vi "Init.vi"(8 "error in (no error)":errorcluster, 11 "Data in":refnum<class "FPGA-Bus.lvclass">) -> (0 "error out":errorcluster, 3 "Data out":refnum<class "FPGA-Bus.lvclass">)   [LabVIEW 2021, in "FPGA-Bus.lvclass"]
doc: "Abstract Data Classes 2.1.1.12\nTim Streeter - TSA\nCopyright (c) 2024, TSAOmni-Bus 2.0.1.6\nTim - TSA\nCopyright (c) 2024, TSA"
uses:
  FPGA-Bus.lvclass
  C:/Program Files (x86)/National Instruments/LabVIEW 2021/vi.lib/TSA/Omni-Bus/Omni-Bus/Bus Access/Bus_Access.lvclass
  <vilib>/TSA/Omni-Bus/Omni-Bus/Bus Access/Bus_Access.lvclass/Bus_Access.ctl
  FPGA-Bus.lvclass/FPGA-Bus.ctl
  Support/Boolean/FPGA-Bus_Boolean.lvclass
  C:/Program Files (x86)/National Instruments/LabVIEW 2021/vi.lib/TSA/Abstract Data Classes/Abs_Types/Value/Abs_Value.lvclass
  Support/Boolean/FPGA-Bus_Boolean.lvclass/FPGA-Bus_Boolean.ctl
  Support/SGL/FPGA-Bus_SGL.lvclass
  Support/SGL/Support/FPGA Type.ctl
  Support/SGL/FPGA-Bus_SGL.lvclass/FPGA-Bus_SGL.ctl
  Support/I8/Support/FPGA Type.ctl
  Support/I8/FPGA-Bus_I8.lvclass
  Support/I8/FPGA-Bus_I8.lvclass/FPGA-Bus_I8.ctl
  Support/I16/Support/FPGA Type.ctl
  Support/I16/FPGA-Bus_I16.lvclass
  Support/I16/FPGA-Bus_I16.lvclass/FPGA-Bus_I16.ctl
  Support/I32/Support/FPGA Type.ctl
  Support/I32/FPGA-Bus_I32.lvclass
  Support/I32/FPGA-Bus_I32.lvclass/FPGA-Bus_I32.ctl
  Support/I64/Support/FPGA Type.ctl
  Support/I64/FPGA-Bus_I64.lvclass
  Support/I64/FPGA-Bus_I64.lvclass/FPGA-Bus_I64.ctl
  Support/U8/Support/FPGA Type.ctl
  Support/U8/FPGA-Bus_U8.lvclass
  Support/U8/FPGA-Bus_U8.lvclass/FPGA-Bus_U8.ctl
  Support/U16/Support/FPGA Type.ctl
  Support/U16/FPGA-Bus_U16.lvclass
  Support/U16/FPGA-Bus_U16.lvclass/FPGA-Bus_U16.ctl
  Support/U32/Support/FPGA Type.ctl
  Support/U32/FPGA-Bus_U32.lvclass
  Support/U32/FPGA-Bus_U32.lvclass/FPGA-Bus_U32.ctl
  Support/U64/Support/FPGA Type.ctl
  Support/U64/FPGA-Bus_U64.lvclass
  Support/U64/FPGA-Bus_U64.lvclass/FPGA-Bus_U64.ctl
  Support/FXP20_5/Support/FPGA Type.ctl
  Support/FXP20_5/FPGA-Bus_FXP20_5.lvclass
  C:/Program Files (x86)/National Instruments/LabVIEW 2021/vi.lib/TSA/Abstract Data Classes/Abs_Types/Double Float/Abs_Double Float.lvclass
  Support/FXP20_5/FPGA-Bus_FXP20_5.lvclass/FPGA-Bus_FXP20_5.ctl
  Support/FXP24_-2/Support/FPGA Type.ctl
  Support/FXP24_-2/FPGA-Bus_FXP24_-2.lvclass
  Support/FXP24_-2/FPGA-Bus_FXP24_-2.lvclass/FPGA-Bus_FXP24_-2.ctl
  Support/FXP24_5/Support/FPGA Type.ctl
  Support/FXP24_5/FPGA-Bus_FXP24_5.lvclass
  Support/FXP24_5/FPGA-Bus_FXP24_5.lvclass/FPGA-Bus_FXP24_5.ctl
  Support/FXP24_10/Support/FPGA Type.ctl
  Support/FXP24_10/FPGA-Bus_FXP24_10.lvclass
  Support/FXP24_10/FPGA-Bus_FXP24_10.lvclass/FPGA-Bus_FXP24_10.ctl
  Support/FXP16_3/Support/FPGA Type.ctl
  Support/FXP16_3/FPGA-Bus_FXP16_3.lvclass
  Support/FXP16_3/FPGA-Bus_FXP16_3.lvclass/FPGA-Bus_FXP16_3.ctl
  Support/FXP18_3/Support/FPGA Type.ctl
  Support/FXP18_3/FPGA-Bus_FXP18_3.lvclass
  Support/FXP18_3/FPGA-Bus_FXP18_3.lvclass/FPGA-Bus_FXP18_3.ctl
  <vilib>/NI/LVFPGA Adv Session Resources/OpenByNameSubVI.vi
  Support/Boolean/Properties/Write FPGA Interface.vi
  Support/SGL/Properties/Write FPGA Interface.vi
  Support/I8/Properties/Write FPGA Interface.vi
  Support/I16/Properties/Write FPGA Interface.vi
  Support/I32/Properties/Write FPGA Interface.vi
  Support/I64/Properties/Write FPGA Interface.vi
  Support/U8/Properties/Write FPGA Interface.vi
  Support/U16/Properties/Write FPGA Interface.vi
  Support/U32/Properties/Write FPGA Interface.vi
  Support/U64/Properties/Write FPGA Interface.vi
  Support/FXP20_5/Properties/Write FPGA Interface.vi
  Support/FXP24_-2/Properties/Write FPGA Interface.vi
  Support/FXP24_5/Properties/Write FPGA Interface.vi
  Support/FXP24_10/Properties/Write FPGA Interface.vi
  Support/FXP16_3/Properties/Write FPGA Interface.vi
  Support/FXP18_3/Properties/Write FPGA Interface.vi
  <vilib>/TSA/Omni-Bus/Omni-Bus/Bus Access/Properties/Read Tag Root.vi
  <vilib>/TSA/Omni-Bus/Omni-Bus/Bus Access/Properties/Write Values.vi
  <vilib>/TSA/Omni-Bus/Omni-Bus/Bus Access/Properties/Write Tags.vi
  <vilib>/TSA/Abstract Data Classes/Abs_Types/Double Float/Abs_Double Float.lvclass
  <vilib>/TSA/Abstract Data Classes/Abs_Types/Value/Abs_Value.lvclass
  C:/Program Files (x86)/National Instruments/LabVIEW 2021/vi.lib/TSA/Abstract Data Classes/Abs_Types/Type/Abs_Type.lvclass
  <vilib>/rvi/interface/common/dynamic/niFpgaEscapeDelimiterAndNull.vi
  <vilib>/Utility/error.llb/Error Cluster From Error Code.vi
  <vilib>/NI/LVFPGA Adv Session Resources/OpenByName.xnode
  <vilib>/NI/LVFPGA Adv Session Resources/LVFPGAAdvSessionResources.lvlib
  <vilib>/Utility/Data Type/NI_Data Type.lvlib
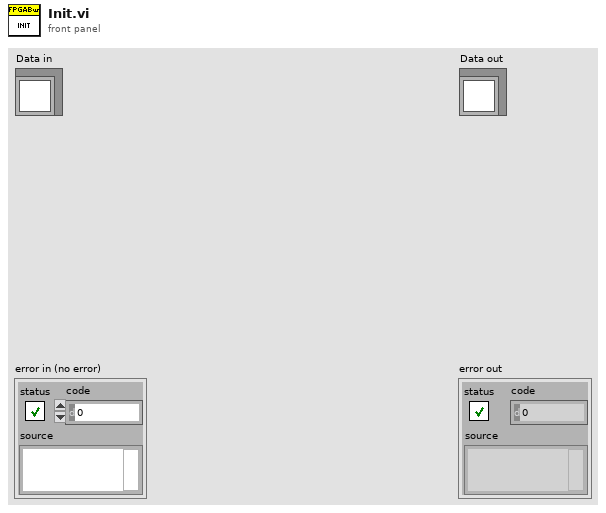
[diagram p1: front panel]
types:
  T1 = typedef "LVFPGAAdvSessionResources.lvlib/ResourceInfo.ctl" = cluster{"Resource name":string, "Data type":variant, "Resource type":enum16{"Register", "Host To Target FIFO", "Target To Host FIFO"}}
  T2 = cluster{"Name":string, "Depth":u32, "Write? (Deprecated:Use Implementation)":bool, "Physical Channel":u32, "Base Address":u32, "Data Width":u32, "Data Type":enum32{"Boolean", "I8", "I16", "I32", "I64", "U8", "U16", "U32", "U64", "FXP", "CustomControl", "SGL"}, "FXP Properties":variant, "Write Window Address":u32, "Implementation":enum16{"niFpgaTargetToHost", "niFpgaHostToTarget", "niFpgaPeerToPeerWriter", "niFpgaPeerToPeerReader", "niCoreTargetToHost", "niCoreHostToTarget"}, "Control Set":u32}[]
  T3 = cluster{"Name":string, "type":variant, "indicator?":bool}[]
  T4 = typedef "FPGA-Bus_SGL.lvclass/FPGA Type.ctl" = refnum<k20>
  T5 = typedef "FPGA-Bus_I8.lvclass/FPGA Type.ctl" = refnum<k20>
  T6 = typedef "FPGA-Bus_I16.lvclass/FPGA Type.ctl" = refnum<k20>
  T7 = typedef "FPGA-Bus_I32.lvclass/FPGA Type.ctl" = refnum<k20>
  T8 = typedef "FPGA-Bus_I64.lvclass/FPGA Type.ctl" = refnum<k20>
  T9 = typedef "FPGA-Bus_U8.lvclass/FPGA Type.ctl" = refnum<k20>
  T10 = typedef "FPGA-Bus_U16.lvclass/FPGA Type.ctl" = refnum<k20>
  T11 = typedef "FPGA-Bus_U32.lvclass/FPGA Type.ctl" = refnum<k20>
  T12 = typedef "FPGA-Bus_U64.lvclass/FPGA Type.ctl" = refnum<k20>
  T13 = typedef "FPGA-Bus_FXP20_5.lvclass/FPGA Type.ctl" = refnum<k20>
  T14 = typedef "FPGA-Bus_FXP24_-2.lvclass/FPGA Type.ctl" = refnum<k20>
  T15 = typedef "FPGA-Bus_FXP24_5.lvclass/FPGA Type.ctl" = refnum<k20>
  T16 = typedef "FPGA-Bus_FXP24_10.lvclass/FPGA Type.ctl" = refnum<k20>
  T17 = typedef "FPGA-Bus_FXP16_3.lvclass/FPGA Type.ctl" = refnum<k20>
  T18 = typedef "FPGA-Bus_FXP18_3.lvclass/FPGA Type.ctl" = refnum<k20>
  T19 = typedef "NI_Data Type.lvlib/Data Type.ctl" = enum8{"Invalid Type", "Void", "I8", "I16", "I32", "I64", "U8", "U16", "U32", "U64", "Single Float", "Double Float", "Extended Float", "Single Complex", "Double Complex", "Extended Complex", "Enum U8", "Enum U16", "Enum U32", "Enum U64", "Single Float With Unit", "Double Float With Unit", "Extended Float With Unit", "Single Complex with Unit", "Double Complex with Unit", "Extended Complex with Unit", "Boolean", "String", "Path", "Picture", "Tag", "Array", "Cluster", "Variant", "LV Variant", "Waveform", "Timestamp", "Digital Waveform", "Digital Data", "ExpressData", "Refnum", "External Data", "VI", "Poly VI", "LabVIEW Class Instance", "Fixed Point", "Set Collection", "Map Collection"}
  T20 = typedef "LVFixedPointRepBitsTypeDef.ctl" = cluster{"Signed":bool, "Word Length":u32, "Integer Word Length":i32}
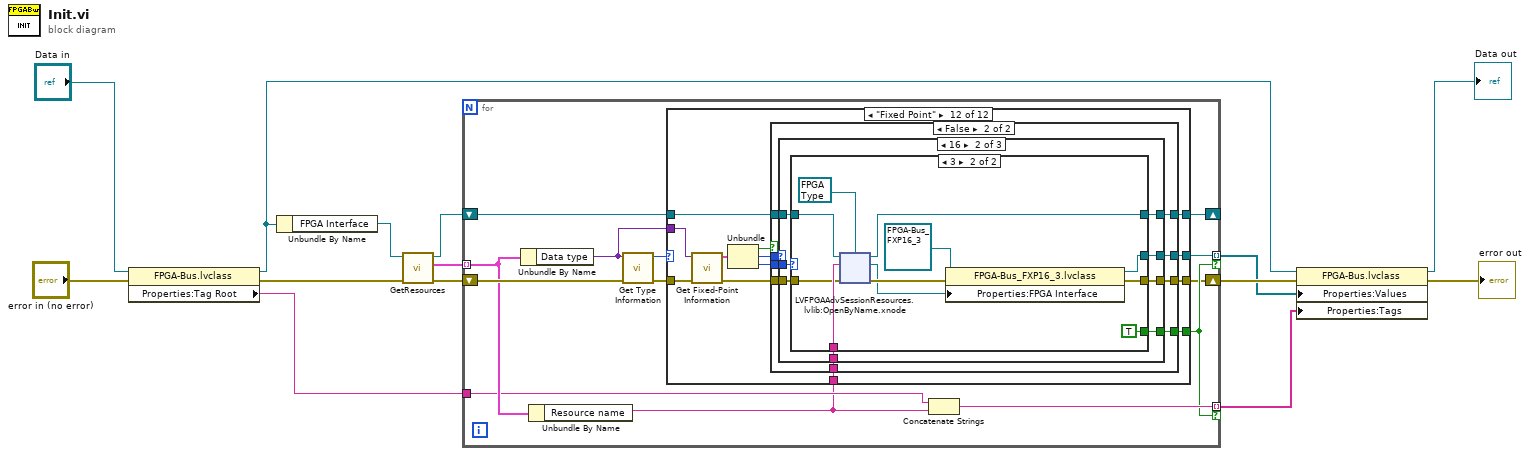
[diagram p0: block diagram]
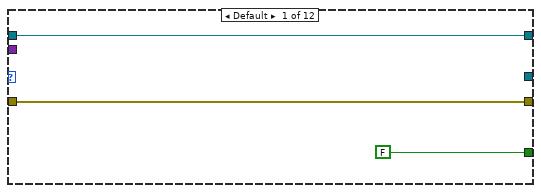
[diagram p2: hidden frame]
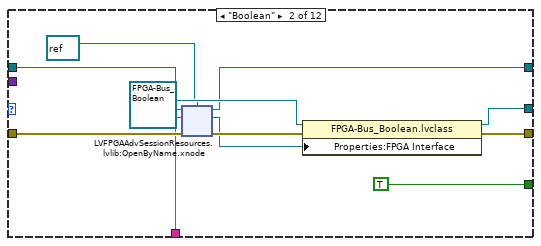
[diagram p3: hidden frame]
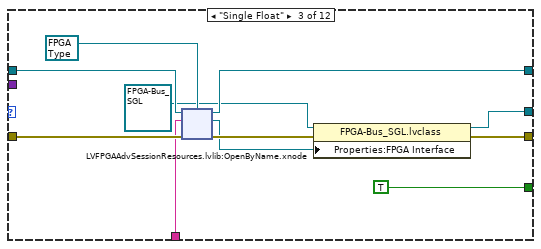
[diagram p4: hidden frame]
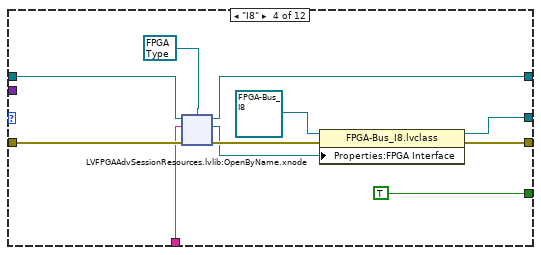
[diagram p5: hidden frame]
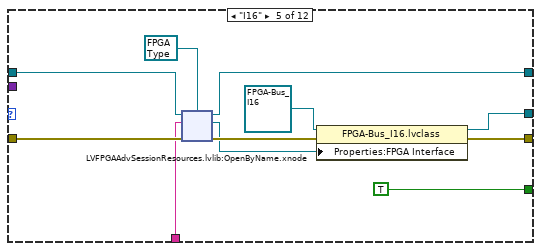
[diagram p6: hidden frame]
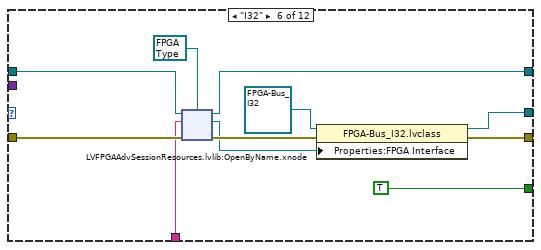
[diagram p7: hidden frame]
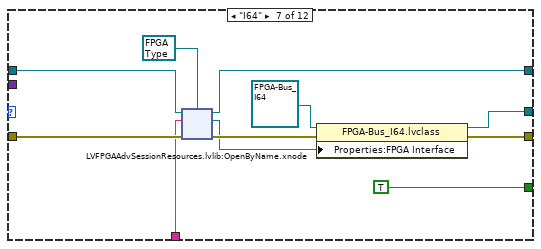
[diagram p8: hidden frame]
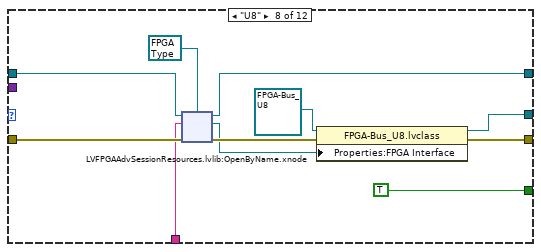
[diagram p9: hidden frame]
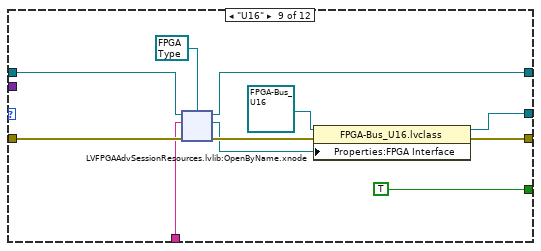
[diagram p10: hidden frame]
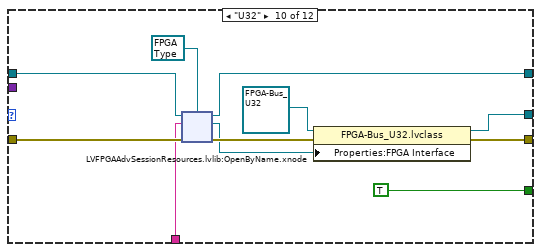
[diagram p11: hidden frame]
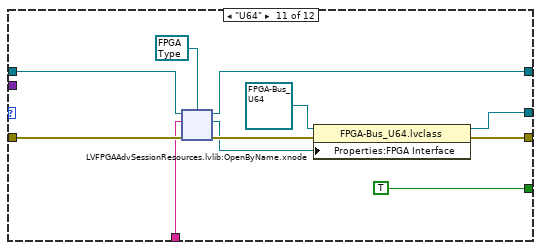
[diagram p12: hidden frame]
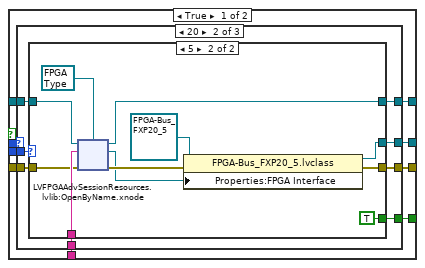
[diagram p13: hidden frame]
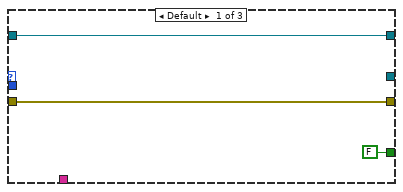
[diagram p14: hidden frame]
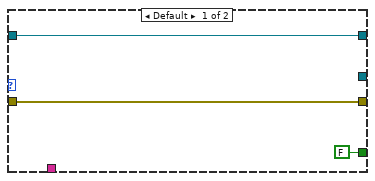
[diagram p15: hidden frame]
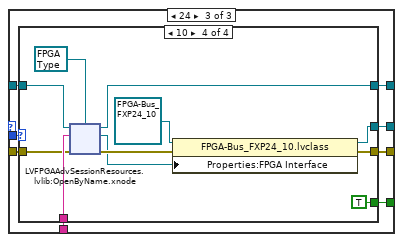
[diagram p16: hidden frame]
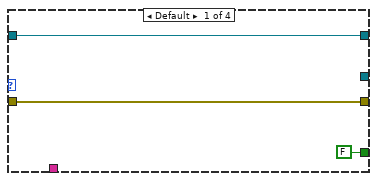
[diagram p17: hidden frame]
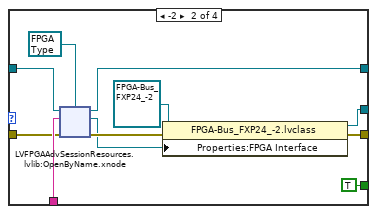
[diagram p18: hidden frame]
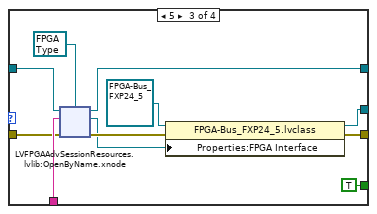
[diagram p19: hidden frame]
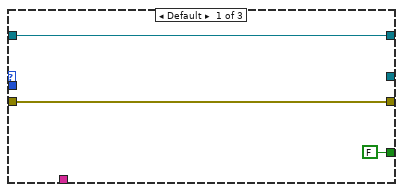
[diagram p20: hidden frame]
diagram:
  n1 = property class="FPGA-Bus.lvclass"(reference="Data in", error in="error in (no error)") -> (reference out=w5:refnum<class "FPGA-Bus.lvclass">, error out=w7:errorcluster, "Properties:Tag Root"=w8:string)
  n2 = Unbundle By Name(w5) -> ("FPGA Interface"=w14:refnum<k20>)
  n3 = call <vilib>:"GetResources.vi"("error in (no error)"=w7, "FPGA VI Reference in"=w14) -> ("error out"=w13:errorcluster, "Resource info out"=w12:T1[], "FPGA VI Reference out"=w11:refnum<k20>)  [unwired: 7 in]
  n4 = for {
    shift-right: [w19] -> w6
    shift-left: w13 -> [w27]
    tunnel: w12 -> [w25] mode=indexing
    tunnel: [w23] -> w4 mode=indexing if=w21
    shift-right: [w16] -> _
    shift-left: w11 -> [w17]
    tunnel: w8 -> [w24]
    tunnel: [w22] -> w1 mode=indexing if=w21
    n5 = Unbundle By Name(w25) -> ("Data type"=w15:variant)
    n6 = Unbundle By Name(w25) -> ("Resource name"=w18:string)
    n7 = call <vilib>:"Get Type Information.vi"("error in (no error)"=w27, "variant"=w15) -> ("error out"=w20:errorcluster, "type"=w26:T19)  [unwired: 5 in, 3 out]
    n8 = case shown="\"Fixed Point\"" w26 {
      tunnel: [FALSE TRUE TRUE TRUE TRUE TRUE TRUE TRUE TRUE TRUE TRUE w283] -> w21
      tunnel: [_ w39 w64 w88 w112 w136 w160 w184 w208 w232 w256 w282] -> w22
      tunnel: w20 -> [w29 w37 w62 w86 w110 w134 w158 w182 w206 w230 w254 w277]
      tunnel: [w29 w38 w63 w87 w111 w135 w159 w183 w207 w231 w255 w281] -> w19
      tunnel: w18 -> [_ w36 w61 w85 w109 w133 w157 w181 w205 w229 w253 w280]
      tunnel: w17 -> [w30 w35 w60 w84 w108 w132 w156 w180 w204 w228 w252 w279]
      tunnel: [w30 w34 w59 w83 w107 w131 w155 w179 w203 w227 w251 w278] -> w16
      tunnel: w15 -> [_ _ _ _ _ _ _ _ _ _ _ w276]
      frame Default {
      }
      frame "Boolean" {
        n9 = xnode "LVFPGAAdvSessionResources.lvlib:OpenByName.xnode"("FPGA VI Reference in"=w35, "Resource name in"=w36, "Single resource reference type in"=refnum<k20> refnum ("FPGA Interface"), "Error in"=w37) -> ("Single resource reference out"=w31:refnum<k20>, "Error out"=w33:errorcluster, "FPGA VI Reference out"=w34:refnum<k20>)
        n10 = property class="FPGA-Bus_Boolean.lvclass"(reference=refnum<class "FPGA-Bus_Boolean.lvclass"> refnum ("FPGA-Bus_Boolean.lvclass"), error in=w33, "Properties:FPGA Interface"=w31) -> (reference out=w39:refnum<class "FPGA-Bus_Boolean.lvclass">, error out=w38:errorcluster)
      }
      frame "Single Float" {
        n11 = xnode "LVFPGAAdvSessionResources.lvlib:OpenByName.xnode"("FPGA VI Reference in"=w60, "Resource name in"=w61, "Single resource reference type in"=T4 refnum ("FPGA Interface"), "Error in"=w62) -> ("Single resource reference out"=w55:T4, "Error out"=w58:errorcluster, "FPGA VI Reference out"=w59:refnum<k20>)
        n12 = property class="FPGA-Bus_SGL.lvclass"(reference=refnum<class "FPGA-Bus_SGL.lvclass"> refnum ("FPGA-Bus_SGL.lvclass"), error in=w58, "Properties:FPGA Interface"=w55) -> (reference out=w64:refnum<class "FPGA-Bus_SGL.lvclass">, error out=w63:errorcluster)
      }
      frame "I8" {
        n13 = xnode "LVFPGAAdvSessionResources.lvlib:OpenByName.xnode"("FPGA VI Reference in"=w84, "Resource name in"=w85, "Single resource reference type in"=T5 refnum ("FPGA Interface"), "Error in"=w86) -> ("Single resource reference out"=w81:T5, "Error out"=w82:errorcluster, "FPGA VI Reference out"=w83:refnum<k20>)
        n14 = property class="FPGA-Bus_I8.lvclass"(reference=refnum<class "FPGA-Bus_I8.lvclass"> refnum ("FPGA-Bus_I8.lvclass"), error in=w82, "Properties:FPGA Interface"=w81) -> (reference out=w88:refnum<class "FPGA-Bus_I8.lvclass">, error out=w87:errorcluster)
      }
      frame "I16" {
        n15 = xnode "LVFPGAAdvSessionResources.lvlib:OpenByName.xnode"("FPGA VI Reference in"=w108, "Resource name in"=w109, "Single resource reference type in"=T6 refnum ("FPGA Interface"), "Error in"=w110) -> ("Single resource reference out"=w105:T6, "Error out"=w106:errorcluster, "FPGA VI Reference out"=w107:refnum<k20>)
        n16 = property class="FPGA-Bus_I16.lvclass"(reference=refnum<class "FPGA-Bus_I16.lvclass"> refnum ("FPGA-Bus_I16.lvclass"), error in=w106, "Properties:FPGA Interface"=w105) -> (reference out=w112:refnum<class "FPGA-Bus_I16.lvclass">, error out=w111:errorcluster)
      }
      frame "I32" {
        n17 = xnode "LVFPGAAdvSessionResources.lvlib:OpenByName.xnode"("FPGA VI Reference in"=w132, "Resource name in"=w133, "Single resource reference type in"=T7 refnum ("FPGA Interface"), "Error in"=w134) -> ("Single resource reference out"=w129:T7, "Error out"=w130:errorcluster, "FPGA VI Reference out"=w131:refnum<k20>)
        n18 = property class="FPGA-Bus_I32.lvclass"(reference=refnum<class "FPGA-Bus_I32.lvclass"> refnum ("FPGA-Bus_I32.lvclass"), error in=w130, "Properties:FPGA Interface"=w129) -> (reference out=w136:refnum<class "FPGA-Bus_I32.lvclass">, error out=w135:errorcluster)
      }
      frame "I64" {
        n19 = xnode "LVFPGAAdvSessionResources.lvlib:OpenByName.xnode"("FPGA VI Reference in"=w156, "Resource name in"=w157, "Single resource reference type in"=T8 refnum ("FPGA Interface"), "Error in"=w158) -> ("Single resource reference out"=w153:T8, "Error out"=w154:errorcluster, "FPGA VI Reference out"=w155:refnum<k20>)
        n20 = property class="FPGA-Bus_I64.lvclass"(reference=refnum<class "FPGA-Bus_I64.lvclass"> refnum ("FPGA-Bus_I64.lvclass"), error in=w154, "Properties:FPGA Interface"=w153) -> (reference out=w160:refnum<class "FPGA-Bus_I64.lvclass">, error out=w159:errorcluster)
      }
      frame "U8" {
        n21 = xnode "LVFPGAAdvSessionResources.lvlib:OpenByName.xnode"("FPGA VI Reference in"=w180, "Resource name in"=w181, "Single resource reference type in"=T9 refnum ("FPGA Interface"), "Error in"=w182) -> ("Single resource reference out"=w177:T9, "Error out"=w178:errorcluster, "FPGA VI Reference out"=w179:refnum<k20>)
        n22 = property class="FPGA-Bus_U8.lvclass"(reference=refnum<class "FPGA-Bus_U8.lvclass"> refnum ("FPGA-Bus_U8.lvclass"), error in=w178, "Properties:FPGA Interface"=w177) -> (reference out=w184:refnum<class "FPGA-Bus_U8.lvclass">, error out=w183:errorcluster)
      }
      frame "U16" {
        n23 = xnode "LVFPGAAdvSessionResources.lvlib:OpenByName.xnode"("FPGA VI Reference in"=w204, "Resource name in"=w205, "Single resource reference type in"=T10 refnum ("FPGA Interface"), "Error in"=w206) -> ("Single resource reference out"=w201:T10, "Error out"=w202:errorcluster, "FPGA VI Reference out"=w203:refnum<k20>)
        n24 = property class="FPGA-Bus_U16.lvclass"(reference=refnum<class "FPGA-Bus_U16.lvclass"> refnum ("FPGA-Bus_U16.lvclass"), error in=w202, "Properties:FPGA Interface"=w201) -> (reference out=w208:refnum<class "FPGA-Bus_U16.lvclass">, error out=w207:errorcluster)
      }
      frame "U32" {
        n25 = xnode "LVFPGAAdvSessionResources.lvlib:OpenByName.xnode"("FPGA VI Reference in"=w228, "Resource name in"=w229, "Single resource reference type in"=T11 refnum ("FPGA Interface"), "Error in"=w230) -> ("Single resource reference out"=w225:T11, "Error out"=w226:errorcluster, "FPGA VI Reference out"=w227:refnum<k20>)
        n26 = property class="FPGA-Bus_U32.lvclass"(reference=refnum<class "FPGA-Bus_U32.lvclass"> refnum ("FPGA-Bus_U32.lvclass"), error in=w226, "Properties:FPGA Interface"=w225) -> (reference out=w232:refnum<class "FPGA-Bus_U32.lvclass">, error out=w231:errorcluster)
      }
      frame "U64" {
        n27 = xnode "LVFPGAAdvSessionResources.lvlib:OpenByName.xnode"("FPGA VI Reference in"=w252, "Resource name in"=w253, "Single resource reference type in"=T12 refnum ("FPGA Interface"), "Error in"=w254) -> ("Single resource reference out"=w249:T12, "Error out"=w250:errorcluster, "FPGA VI Reference out"=w251:refnum<k20>)
        n28 = property class="FPGA-Bus_U64.lvclass"(reference=refnum<class "FPGA-Bus_U64.lvclass"> refnum ("FPGA-Bus_U64.lvclass"), error in=w250, "Properties:FPGA Interface"=w249) -> (reference out=w256:refnum<class "FPGA-Bus_U64.lvclass">, error out=w255:errorcluster)
      }
      frame "Fixed Point" {
        n29 = call <vilib>:"Get Fixed-Point Information.vi"("error in (no error)"=w277, "variant"=w276) -> ("error out"=w273:errorcluster, "FXP representation"=w275:T20)  [unwired: 6 in, 2 out]
        n30 = Unbundle(w275) -> ("Signed"=w274:bool, "Word Length"=w272:u32, "Integer Word Length"=w271:i32)
        n31 = case shown="False" w274 {
          tunnel: [w292 w422] -> w283
          tunnel: [w291 w421] -> w282
          tunnel: [w290 w420] -> w281
          tunnel: w280 -> [w289 w419]
          tunnel: w279 -> [w288 w418]
          tunnel: [w287 w417] -> w278
          tunnel: w273 -> [w286 w416]
          tunnel: w272 -> [w285 w415]
          tunnel: w271 -> [w284 w414]
          frame True {
            n32 = case shown="20" w285 {
              tunnel: [FALSE w303 w338] -> w292
              tunnel: [_ w302 w337] -> w291
              tunnel: [w294 w301 w336] -> w290
              tunnel: w289 -> [_ w300 w335]
              tunnel: w288 -> [w295 w299 w334]
              tunnel: [w295 w298 w333] -> w287
              tunnel: w286 -> [w294 w297 w332]
              tunnel: w284 -> [_ w296 w331]
              frame Default {
              }
              frame 20 {
                n33 = case shown="5" w296 {
                  tunnel: [FALSE TRUE] -> w303
                  tunnel: [_ w316] -> w302
                  tunnel: [w305 w315] -> w301
                  tunnel: w300 -> [_ w314]
                  tunnel: w299 -> [w306 w313]
                  tunnel: [w306 w312] -> w298
                  tunnel: w297 -> [w305 w309]
                  frame Default {
                  }
                  frame 5 {
                    n34 = xnode "LVFPGAAdvSessionResources.lvlib:OpenByName.xnode"("FPGA VI Reference in"=w313, "Resource name in"=w314, "Single resource reference type in"=T13 refnum ("FPGA Interface"), "Error in"=w309) -> ("Single resource reference out"=w310:T13, "Error out"=w311:errorcluster, "FPGA VI Reference out"=w312:refnum<k20>)
                    n35 = property class="FPGA-Bus_FXP20_5.lvclass"(reference=refnum<class "FPGA-Bus_FXP20_5.lvclass"> refnum ("FPGA-Bus_FXP20_5.lvclass"), error in=w311, "Properties:FPGA Interface"=w310) -> (reference out=w316:refnum<class "FPGA-Bus_FXP20_5.lvclass">, error out=w315:errorcluster)
                  }
                }
              }
              frame 24 {
                n36 = case shown="10" w331 {
                  tunnel: [FALSE TRUE TRUE TRUE] -> w338
                  tunnel: [_ w351 w375 w399] -> w337
                  tunnel: [w340 w350 w374 w398] -> w336
                  tunnel: w335 -> [_ w349 w373 w397]
                  tunnel: w334 -> [w341 w348 w372 w396]
                  tunnel: [w341 w347 w371 w395] -> w333
                  tunnel: w332 -> [w340 w344 w368 w392]
                  frame Default {
                  }
                  frame -2 {
                    n37 = xnode "LVFPGAAdvSessionResources.lvlib:OpenByName.xnode"("FPGA VI Reference in"=w348, "Resource name in"=w349, "Single resource reference type in"=T14 refnum ("FPGA Interface"), "Error in"=w344) -> ("Single resource reference out"=w345:T14, "Error out"=w346:errorcluster, "FPGA VI Reference out"=w347:refnum<k20>)
                    n38 = property class="FPGA-Bus_FXP24_-2.lvclass"(reference=refnum<class "FPGA-Bus_FXP24_-2.lvclass"> refnum ("FPGA-Bus_FXP24_-2.lvclass"), error in=w346, "Properties:FPGA Interface"=w345) -> (reference out=w351:refnum<class "FPGA-Bus_FXP24_-2.lvclass">, error out=w350:errorcluster)
                  }
                  frame 5 {
                    n39 = xnode "LVFPGAAdvSessionResources.lvlib:OpenByName.xnode"("FPGA VI Reference in"=w372, "Resource name in"=w373, "Single resource reference type in"=T15 refnum ("FPGA Interface"), "Error in"=w368) -> ("Single resource reference out"=w369:T15, "Error out"=w370:errorcluster, "FPGA VI Reference out"=w371:refnum<k20>)
                    n40 = property class="FPGA-Bus_FXP24_5.lvclass"(reference=refnum<class "FPGA-Bus_FXP24_5.lvclass"> refnum ("FPGA-Bus_FXP24_5.lvclass"), error in=w370, "Properties:FPGA Interface"=w369) -> (reference out=w375:refnum<class "FPGA-Bus_FXP24_5.lvclass">, error out=w374:errorcluster)
                  }
                  frame 10 {
                    n41 = xnode "LVFPGAAdvSessionResources.lvlib:OpenByName.xnode"("FPGA VI Reference in"=w396, "Resource name in"=w397, "Single resource reference type in"=T16 refnum ("FPGA Interface"), "Error in"=w392) -> ("Single resource reference out"=w393:T16, "Error out"=w394:errorcluster, "FPGA VI Reference out"=w395:refnum<k20>)
                    n42 = property class="FPGA-Bus_FXP24_10.lvclass"(reference=refnum<class "FPGA-Bus_FXP24_10.lvclass"> refnum ("FPGA-Bus_FXP24_10.lvclass"), error in=w394, "Properties:FPGA Interface"=w393) -> (reference out=w399:refnum<class "FPGA-Bus_FXP24_10.lvclass">, error out=w398:errorcluster)
                  }
                }
              }
            }
          }
          frame False {
            n43 = case shown="16" w415 {
              tunnel: [FALSE w433 w468] -> w422
              tunnel: [_ w432 w467] -> w421
              tunnel: [w424 w431 w466] -> w420
              tunnel: w419 -> [_ w430 w465]
              tunnel: w418 -> [w425 w429 w464]
              tunnel: [w425 w428 w463] -> w417
              tunnel: w416 -> [w424 w427 w462]
              tunnel: w414 -> [_ w426 w461]
              frame Default {
              }
              frame 16 {
                n44 = case shown="3" w426 {
                  tunnel: [FALSE TRUE] -> w433
                  tunnel: [_ w446] -> w432
                  tunnel: [w435 w445] -> w431
                  tunnel: w430 -> [_ w444]
                  tunnel: w429 -> [w436 w443]
                  tunnel: [w436 w442] -> w428
                  tunnel: w427 -> [w435 w439]
                  frame Default {
                  }
                  frame 3 {
                    n45 = xnode "LVFPGAAdvSessionResources.lvlib:OpenByName.xnode"("FPGA VI Reference in"=w443, "Resource name in"=w444, "Single resource reference type in"=T17 refnum ("FPGA Interface"), "Error in"=w439) -> ("Single resource reference out"=w440:T17, "Error out"=w441:errorcluster, "FPGA VI Reference out"=w442:refnum<k20>)
                    n46 = property class="FPGA-Bus_FXP16_3.lvclass"(reference=refnum<class "FPGA-Bus_FXP16_3.lvclass"> refnum ("FPGA-Bus_FXP16_3.lvclass"), error in=w441, "Properties:FPGA Interface"=w440) -> (reference out=w446:refnum<class "FPGA-Bus_FXP16_3.lvclass">, error out=w445:errorcluster)
                  }
                }
              }
              frame 18 {
                n47 = case shown="3" w461 {
                  tunnel: [FALSE TRUE] -> w468
                  tunnel: [_ w481] -> w467
                  tunnel: [w470 w480] -> w466
                  tunnel: w465 -> [_ w479]
                  tunnel: w464 -> [w471 w478]
                  tunnel: [w471 w477] -> w463
                  tunnel: w462 -> [w470 w474]
                  frame Default {
                  }
                  frame 3 {
                    n48 = xnode "LVFPGAAdvSessionResources.lvlib:OpenByName.xnode"("FPGA VI Reference in"=w478, "Resource name in"=w479, "Single resource reference type in"=T18 refnum ("FPGA Interface"), "Error in"=w474) -> ("Single resource reference out"=w475:T18, "Error out"=w476:errorcluster, "FPGA VI Reference out"=w477:refnum<k20>)
                    n49 = property class="FPGA-Bus_FXP18_3.lvclass"(reference=refnum<class "FPGA-Bus_FXP18_3.lvclass"> refnum ("FPGA-Bus_FXP18_3.lvclass"), error in=w476, "Properties:FPGA Interface"=w475) -> (reference out=w481:refnum<class "FPGA-Bus_FXP18_3.lvclass">, error out=w480:errorcluster)
                  }
                }
              }
            }
          }
        }
      }
    }
    n50 = Concatenate Strings(w24, w18) -> (w23:string)
  }
  n51 = property class="FPGA-Bus.lvclass"(reference=w5, error in=w6, "Properties:Values"=w1, "Properties:Tags"=w4) -> (reference out=→"Data out":refnum<class "FPGA-Bus.lvclass">, error out=→"error out":errorcluster)
